vi "Read Plugin Settings ID.vi"(8 "error in (no error)":errorcluster, 10 "Plugin ID":string, 11 "dsf refnum":T1) -> (0 "error out":errorcluster, 1 "Settings ID":string, 3 "dsf refnum out":T1, 4 "found?":bool)   [LabVIEW 2017, in "DSF Core.lvlib"]
uses:
  DSF Core.lvlib
  Controls/DSF Config Data RefNum.ctl
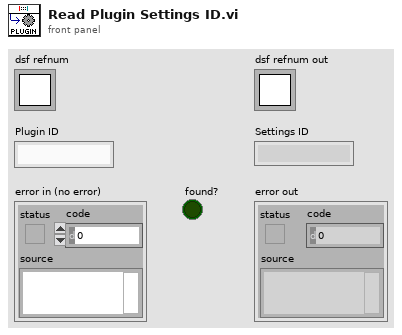
[diagram p1: front panel]
types:
  T1 = typedef "DSF Core.lvlib/DSF Config Data RefNum.ctl" = refnum<k1>
  T2 = typedef "DSF Core.lvlib/DSF Configuration Reference.ctl" = refnum<data-value>
  T3 = typedef "DSF Core.lvlib/Internal.DSF Configuration.ctl" = cluster{"dsfversion":T4, "version":T4, "plugins":T5[], "groups":T8[], "transfers":T10[], "channels":T12[], "settings":T14[]}
  T4 = typedef "DSF Core.lvlib/DSF Version Info.ctl" = cluster{"major":u32, "minor":u32, "fix":u32, "build":string}
  T5 = typedef "DSF Core.lvlib/Internal.DSF Plugin with ID.ctl" = cluster{"id":string, "values":T6}
  T6 = typedef "DSF Core.lvlib/Internal.DSF Plugin Info.ctl" = cluster{"type":string, "timing":T7, "group ids":string[], "settings id":string}
  T7 = typedef "DSF Core.lvlib/DSF Timing Info.ctl" = cluster{"priority":u64, "decimation":u64, "offset":u64}
  T8 = typedef "DSF Core.lvlib/Internal.DSF Group with ID.ctl" = cluster{"id":string, "values":T9}
  T9 = typedef "DSF Core.lvlib/Internal.DSF Group Info.ctl" = cluster{"direction":i32, "timing":T7, "transfer ids":string[], "settings id":string}
  T10 = typedef "DSF Core.lvlib/Internal.DSF Transfer with ID.ctl" = cluster{"id":string, "values":T11}
  T11 = typedef "DSF Core.lvlib/Internal.DSF Transfer Info.ctl" = cluster{"byte order":i32, "channel ids":string[], "settings id":string}
  T12 = typedef "DSF Core.lvlib/Internal.DSF Channel with ID.ctl" = cluster{"id":string, "values":T13}
  T13 = typedef "DSF Core.lvlib/Internal.DSF Channel Info.ctl" = cluster{"count":u64, "buffer offset":u64, "data type":i32, "settings id":string}
  T14 = typedef "DSF Core.lvlib/Internal.DSF Settings with ID.ctl" = cluster{"id":string, "values":T15}
  T15 = typedef "DSF Core.lvlib/Internal.DSF Settings Info.ctl" = cluster{"key":string, "value":string}[]
  T16 = cluster{"dsf configuration":T3, "path":path, "dirty":bool}
  T17 = typedef "DSF Core.lvlib/DSF Plugin Info.ctl" = cluster{"type":string, "timing":T7, "group ids":string[], "settings id":string}
  T18 = typedef "DSF Core.lvlib/DSF Config Data.ctl" = cluster{"dsf configuration":T3, "path":path, "dirty":bool}
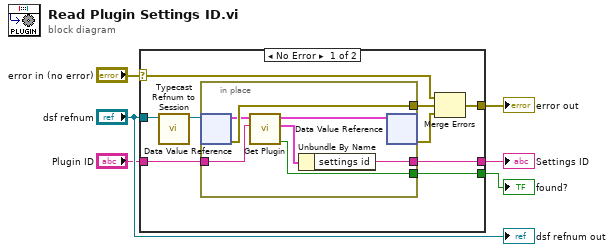
[diagram p0: block diagram]
diagram:
  n1 = case shown="No Error" "error in (no error)" {
    selector: "error in (no error)" -> [w15 w23]
    tunnel: "dsf refnum" -> [w14 _]
    tunnel: [w11 w23] -> w4
    tunnel: "Plugin ID" -> [w13 _]
    tunnel: [w8 _] -> w2
    tunnel: [w7 _] -> w1
    frame No Error {
      n2 = call "Typecast Refnum to Session.vi"("dsf refnum in"=w14) -> ("DSF Configuration Session out"=w12:T2)  [unwired: 10 in]
      n3 = in-place {
        in-place-border: w13 -> [w20]
        in-place-border: [w22] -> w10
        in-place-border: [w19] -> w8
        in-place-border: [w16] -> w7
        n4 = in-place-dvr #1(w12) -> (w21:T16, w22:errorcluster)
        n5 = call "Get Plugin.vi"("id"=w20, "DSF Configuration in"=w21) -> ("exists?"=w19:bool, "info"=w17:T17, "DSF Configuration out"=w18:T18)  [unwired: 6 in, 1 out]
        n6 = Unbundle By Name(w17) -> ("settings id"=w16:string)
        n7 = in-place-dvr #1(w18) -> (w9:errorcluster)  [unwired: 1 out]
      }
      n8 = Merge Errors(w15, w10, w9) -> (w11:errorcluster)
    }
    frame Error {
    }
  }
  "error out" <- w4
  "found?" <- w2
  "Settings ID" <- w1
  "dsf refnum out" <- "dsf refnum"
